vi "BigCryoT.vi"() -> ()   [LabVIEW 2019]
uses:
  <vilib>/Instr/_visa.llb/VISA Configure Serial Port (Instr).vi
panel:
  in  "Termination Character":u8=10 format="%.0x"
  out "read buffer":string
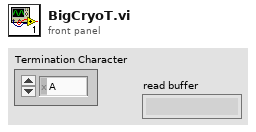
[diagram p1: front panel]
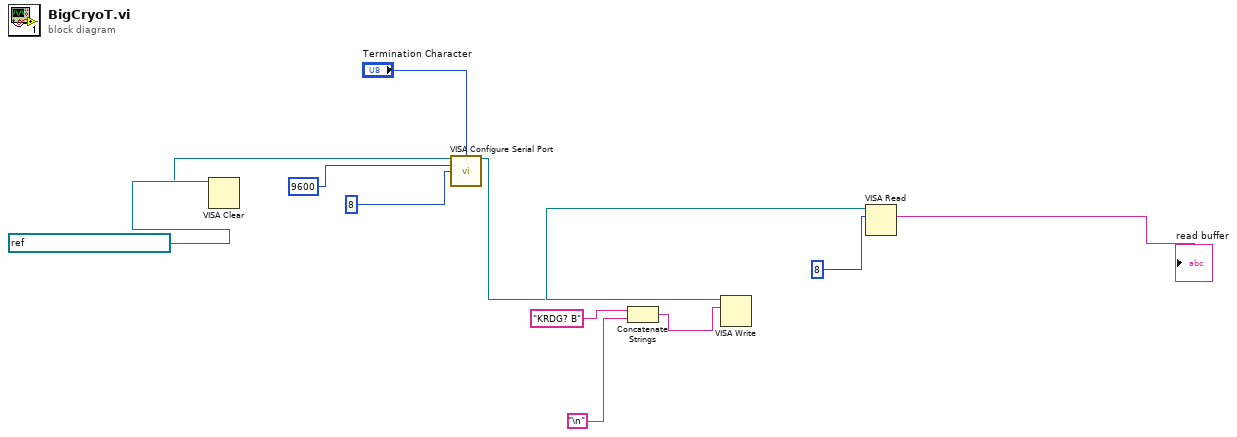
[diagram p0: block diagram]
diagram:
  n1 = VISA Clear(VISA resource name=refnum<visa-resource-name> "COM7") -> (VISA resource name out=w3:refnum<visa-resource-name>)  [unwired: 1 in, 1 out]
  n2 = call-poly "VISA Configure Serial Port"("VISA resource name"=w3, "termination char\n(0xA = '\\n' = LF)"="Termination Character", "baud rate (9600)"=9600, "data bits (8)"=8) -> ("VISA resource name out"=w7:refnum<visa-resource-name>)  [unwired: 10 in, 1 out]
  n3 = Concatenate Strings("KRDG? B" ("write buffer"), "\n") -> (w1:string)
  n4 = VISA Write(VISA resource name=w7, write buffer=w1) -> (VISA resource name out=w10:refnum<visa-resource-name>)  [unwired: 1 in, 2 out]
  n5 = VISA Read(VISA resource name=w10, byte count=u32 8) -> (read buffer=→"read buffer":string)  [unwired: 1 in, 3 out]
